vi "solar_voy_def Import (Variant).vi"(4 "Default ID":u16, 5 "Endian (BIG)":enum8{"BIG", "LITTLE"}(ring), 6 "Suppress Errors? (T)":bool=TRUE, 7 "CMD":enum8{"CMD", "TLM"}(ring), 8 "error in (no error)":errorcluster, 9 "Variant":variant, 10 "PACKET (\"\"=Use Variant)":string, 11 "TARGET":string) -> (0 "error out":errorcluster, 3 "PACKET":T1 {"last_time" format="%<%H:%M:%S%3u %m/%d/%y>T"})   [LabVIEW 2018]
doc: "This imports a Voyager packet definition from a LabVIEW variant. The variant should be a cluster packet, and elements for each parameter/item. Use the followin arguments to modify each parameter/item via the label as '<label>,<arg0>,<arg1>'.\n\nLabel Modifiers:\nt=TYPE (block|string|int|uint|float) - Sets the COSMOS data type\nlv=LVTYPE (u8..u64,i8..i64,sgl,dbl,string,boolean,u16_enum,etc.) - Sets the LabVIEW data type\nb=BIT_SIZE - Sets the total parameter/item bit size\ne=EACH_BIT_SIZE - Sets the element bit size for string or block arrays only\ns=STATE|STATE - Sets the states starting at value 0:STATE|1:STATE|etc.\nid - Sets the ID flag\nd=DESC - Sets the item's description. Must be set at end of labels\n\nExamples: \nMYBLOCKARRAY,t=block,lv=string,b=64,e=16 # 1D array of U16 blocks of 4 elements (64 bits / 16 each) \nMYU16KEY,t=uint,lv=u16,b=16,id # U16 id parameter\nMYBOOLEAN,t=uint,lv=boolean,b=1,s=OK|ERROR # 1 bit boolean with false:OK, true:ERROR states"
uses:
  type/solar_type Item Type.ctl
  solar_voy_def_ctl ITEM TYPE.ctl
  solar_voy_def_ctl MODIFIERS CONVERSION.ctl
  solar_voy_def_ctl MODIFIERS STATE.ctl
  solar_voy_def_ctl MODIFIERS UNITS.ctl
  solar_voy_def_ctl MODIFIERS LIMITS.ctl
  solar_voy_def_ctl MODIFIERS.ctl
  solar_voy_def_ctl ITEM.ctl
  solar_voy_def_ctl PACKET.ctl
  solar_voy_def_ctl PACKET_ID.ctl
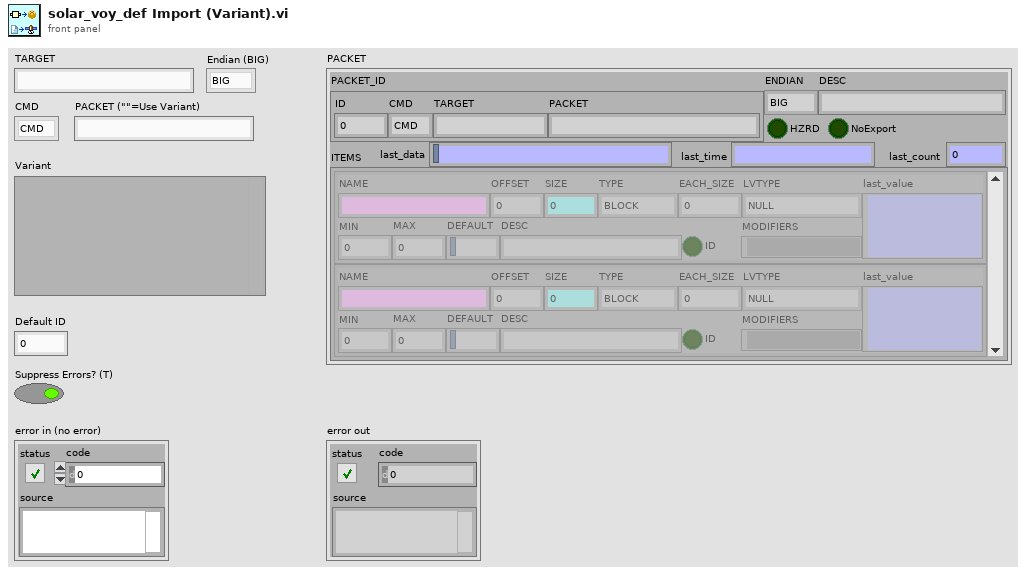
[diagram p1: front panel]
types:
  T1 = typedef "solar_voy_def_ctl PACKET.ctl" = cluster{"PACKET_ID":T2, "ENDIAN":enum8{"BIG", "LITTLE"}, "DESC":string, "HZRD":bool, "ITEMS":T3[], "NoExport":bool, "last_time":timestamp, "last_count":u32, "last_data":string}
  T2 = typedef "solar_voy_def_ctl PACKET_ID.ctl" = cluster{"ID":u16, "CMD":enum8{"CMD", "TLM"}, "TARGET":string, "PACKET":string}
  T3 = typedef "solar_voy_def_ctl ITEM.ctl" = cluster{"NAME":string, "OFFSET":i32, "SIZE":i32, "TYPE":T4, "EACH_SIZE":i32, "LVTYPE":T5, "MIN":dbl, "MAX":dbl, "DEFAULT":string, "DESC":string, "ID":bool, "MODIFIERS":variant, "last_value":variant}
  T4 = typedef "solar_voy_def_ctl ITEM TYPE.ctl" = enum8{"BLOCK", "INT", "UINT", "FLOAT", "STRING"}
  T5 = typedef "solar_type Item Type.ctl" = enum16{"NULL", "UNKNOWN", "CLUSTER", "I8", "I16", "I32", "I64", "U8", "U16", "U32", "U64", "U8_ENUM", "U16_ENUM", "U32_ENUM", "SGL", "DBL", "BOOLEAN", "STRING", "PATH", "VISA", "TAG", "TIME", "I8_1D", "I16_1D", "I32_1D", "I64_1D", "U8_1D", "U16_1D", "U32_1D", "U64_1D", "U8_ENUM_1D", "U16_ENUM_1D", "U32_ENUM_1D", "SGL_1D", "DBL_1D", "BOOLEAN_1D", "STRING_1D", "PATH_1D", "VISA_1D", "TAG_1D", "TIME_1D", "I8_2D", "I16_2D", "I32_2D", "I64_2D", "U8_2D", "U16_2D", "U32_2D", "U64_2D", "U8_ENUM_2D", "U16_ENUM_2D", "U32_ENUM_2D", "SGL_2D", "DBL_2D", "BOOLEAN_2D", "STRING_2D", "PATH_2D", "VISA_2D", "TAG_2D", "TIME_2D"}
  T6 = typedef "solar_type Item.ctl" = cluster{"Item":string, "Type":T5, "Value":variant, "States":string[]}
  T7 = typedef "solar_voy_def_ctl MODIFIERS.ctl" = cluster{"LIMITS":T8, "UNITS":T9, "STATES":T10[], "CONVERSION":T11, "FORMAT":string, "REQUIRED":bool, "META":string[][]}
  T8 = typedef "solar_voy_def_ctl MODIFIERS LIMITS.ctl" = cluster{"NAME":string, "PERSIST":i32, "EN":bool, "RED_LO":dbl, "YEL_LO":dbl, "YEL_HI":dbl, "RED_HI":dbl, "GRN_LO":dbl, "GRN_HI":dbl, "FILENAME":string, "ARGS":string}
  T9 = typedef "solar_voy_def_ctl MODIFIERS UNITS.ctl" = cluster{"FULL":string, "ABV":string}
  T10 = typedef "solar_voy_def_ctl MODIFIERS STATE.ctl" = cluster{"KEY":string, "VALUE":string, "COLOR":string, "DESC":string, "HZRD":bool}
  T11 = typedef "solar_voy_def_ctl MODIFIERS CONVERSION.ctl" = cluster{"GENERIC":string, "FILENAME":string, "ARGS":string, "POLYS":cluster{"SEG":bool, "POLY":dbl[]}[]}
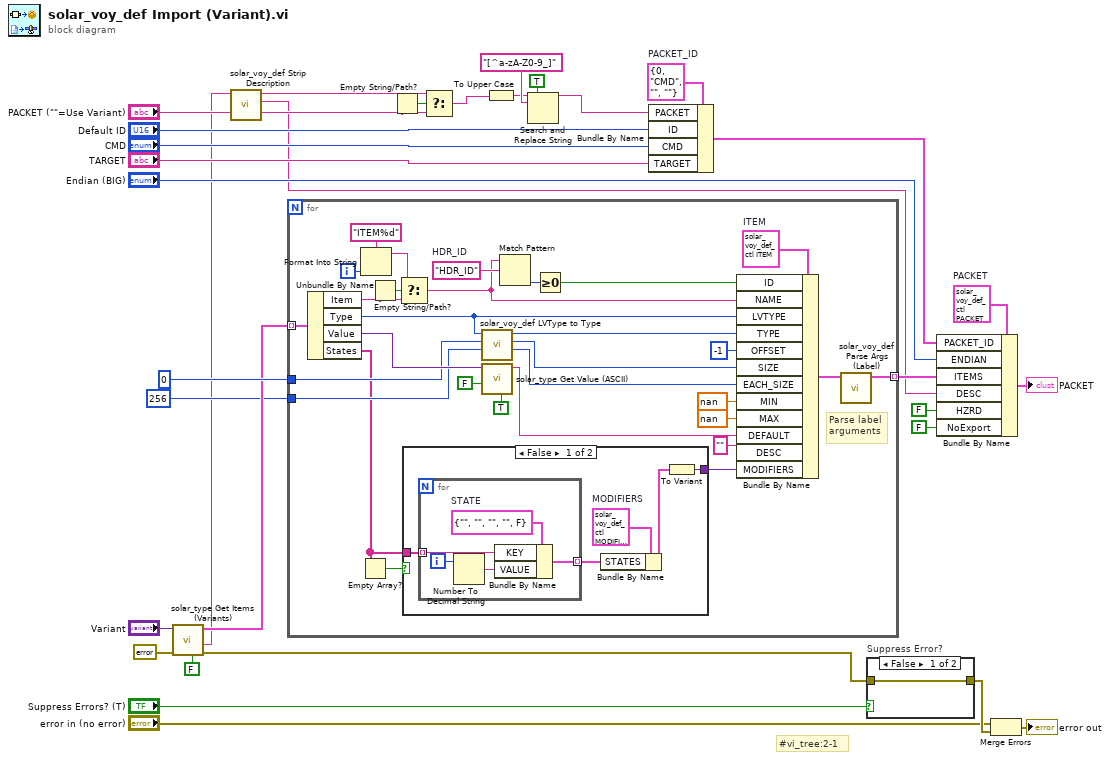
[diagram p0: block diagram]
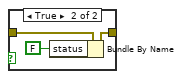
[diagram p3: hidden frame]
diagram:
  w13 = T2 {"ID"=0, "CMD"=enum."CMD", "TARGET"="", "PACKET"=""}  # PACKET_ID
  w16 = T1 {"PACKET_ID"={"ID"=0, "CMD"=enum."CMD", "TARGET"="", "PACKET"=""}, "ENDIAN"=enum."BIG", "DESC"="", "HZRD"=FALSE, "ITEMS"=[], "NoExport"=FALSE, "last_time"=timestamp(0 s since 1904-01-01), "last_count"=0, "last_data"=""}  # PACKET
  # "#vi_tree:2-1"
  n1 = call "solar_type Get Items (Variants).vi"("Include Cluster Prefix? (F)"=FALSE, "error in (no error)"=errorcluster {"status"=FALSE, "code"=0, "source"=""}, "Variant"="Variant") -> ("error out"=w29:errorcluster, "Variant Name"=w3:string, "Items"=w19:T6[])  [unwired: 5 in, 1 out]
  n2 = call "solar_voy_def Strip Description.vi"("Name String"=w3) -> ("Description"=w1:string, "Fixed Name"=w2:string)  [unwired: 9 in]
  n3 = for {
    tunnel: [w50] -> w15 mode=indexing
    tunnel: w19 -> [w62] mode=indexing
    tunnel: 0 ("Variable Size (0 bits = rest)") -> [w52]
    tunnel: 256 ("Each Array Item (256 bits) [1D Str only]") -> [w51]
    i -> [w59]
    w40 = T3 {"NAME"="", "OFFSET"=0, "SIZE"=0, "TYPE"=enum."BLOCK", "EACH_SIZE"=0, "LVTYPE"=enum."NULL", "MIN"=0.0, "MAX"=0.0, "DEFAULT"="", "DESC"="", "ID"=FALSE, "MODIFIERS"=variant, "last_value"=variant}  # ITEM
    w57 = "HDR_ID"  # HDR_ID
    # "Parse label\narguments"
    n4 = Unbundle By Name(w62) -> ("Item"=w48:string, "Type"=w45:T5, "Value"=w55:variant, "States"=w34:string[])
    n5 = Empty Array?(array=w34) -> (empty?=w33:bool)
    n6 = Format Into String(format string="ITEM%d", w59) -> (resulting string=w60:string)  [unwired: 2 in, 1 out]
    n7 = Empty String/Path?(string/path=w48) -> (empty?=w61:bool)
    n8 = Select(t=w60, s=w61, f=w48) -> (s? t:f=w47:string)
    n9 = case shown="False" w33 {
      tunnel: w34 -> [w64 _]
      tunnel: [w63 _] -> w35
      frame False {
        w65 = T7 {"LIMITS"={"NAME"="", "PERSIST"=0, "EN"=FALSE, "RED_LO"=0.0, "YEL_LO"=0.0, "YEL_HI"=0.0, "RED_HI"=0.0, "GRN_LO"=0.0, "GRN_HI"=0.0, "FILENAME"="", "ARGS"=""}, "UNITS"={"FULL"="", "ABV"=""}, "STATES"=[], "CONVERSION"={"GENERIC"="", "FILENAME"="", "ARGS"="", "POLYS"=[]}, "FORMAT"="", "REQUIRED"=FALSE, "META"=[]}  # MODIFIERS
        n10 = for {
          tunnel: [w71] -> w67 mode=indexing
          tunnel: w64 -> [w68] mode=indexing
          i -> [w70]
          w72 = T10 {"KEY"="", "VALUE"="", "COLOR"="", "DESC"="", "HZRD"=FALSE}  # STATE
          n11 = Number To Decimal String(number=w70) -> (decimal integer string=w69:string)  [unwired: 1 in]
          n12 = Bundle By Name(cluster=w72, "KEY"=w68, "VALUE"=w69) -> (w71:T10)
        }
        n13 = Bundle By Name(cluster=w65, "STATES"=w67) -> (w66:T7)
        n14 = To Variant(anything=w66) -> (Variant=w63:variant)
      }
      frame True {
      }
    }
    n15 = call "solar_voy_def LVType to Type.vi"("Each Array Item (256 bits) [1D Str only]"=w51, "Variable Size (0 bits = rest)"=w52, "LVTYPE"=w45) -> ("EACH_SIZE (0=NoArray)"=w37:i32, "TOTAL_SIZE (0)"=w46:i32, "TYPE (BLOCK)"=w39:T4)  [unwired: 6 in]
    n16 = call "solar_type Get Value (ASCII).vi"("Boolean as 0,1? (F)"=TRUE, "Use Enum Names? (F)"=FALSE, "Variant"=w55) -> ("Value (ASCII)"=w44:string)  [unwired: 6 in, 2 out]
    n17 = Match Pattern(string=w47, regular expression=w57) -> (offset past match=w56:i32)  [unwired: 1 in, 3 out]
    n18 = Greater Or Equal To 0?(x=w56) -> (x >= 0?=w36:bool)
    n19 = Bundle By Name(cluster=w40, "ID"=w36, "NAME"=w47, "LVTYPE"=w45, "TYPE"=w39, "OFFSET"=-1, "SIZE"=w46, "EACH_SIZE"=w37, "MIN"=nan, "MAX"=nan, "DEFAULT"=w44, "DESC"="", "MODIFIERS"=w35) -> (w49:T3)
    n20 = call "solar_voy_def Parse Args (Label).vi"("Default ITEM"=w49) -> ("ITEM out"=w50:T3)  [unwired: 10 in]
  }
  n21 = Empty String/Path?(string/path="PACKET (\"\"=Use Variant)") -> (empty?=w14:bool)
  n22 = Select(t=w2, s=w14, f="PACKET (\"\"=Use Variant)") -> (s? t:f=w5:string)
  n23 = To Upper Case(1:w5) -> (0:w6:string)
  n24 = Search and Replace String(replace all?=TRUE, input string=w6, search string="[^a-zA-Z0-9_]") -> (result string=w4:string)  [unwired: 5 in, 3 out]
  n25 = Bundle By Name(cluster=w13, "PACKET"=w4, "ID"="Default ID", "CMD"="CMD", "TARGET"="TARGET") -> (w9:T2)
  n26 = case "Suppress Error?" shown="False" "Suppress Errors? (T)" {
    tunnel: w29 -> [w73 w76]
    tunnel: [w73 w75] -> w30
    frame False {
    }
    frame True {
      n27 = Bundle By Name(cluster=w76, "status"=FALSE) -> (w75:errorcluster)
    }
  }
  n28 = Bundle By Name(cluster=w16, "PACKET_ID"=w9, "ENDIAN"="Endian (BIG)", "ITEMS"=w15, "DESC"=w1, "HZRD"=FALSE, "NoExport"=FALSE) -> (→"PACKET":T1)
  n29 = Merge Errors("error in (no error)", w30) -> (→"error out":errorcluster)
